vi "Enqueue Message.vi"(6 "Prioritary message":bool, 7 "QueueName":string, 8 "error in":errorcluster, 9 "Data":variant, 10 "Message":string, 11 "Queue":refnum<queue>) -> (0 "error out":errorcluster, 3 "Queue dup.":refnum<queue>)   [LabVIEW 2016, in "Message Queue.lvlib"]
doc: "Pour un message normal, placer le message à la fin de la file d'attente. Pour un message prioritaire, l'ajouter au début de la file."
uses:
  Message Queue.lvlib
  Message Cluster.ctl
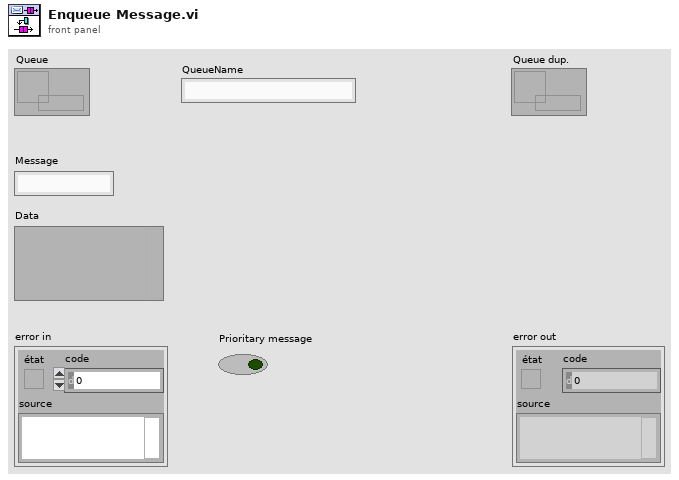
[diagram p1: front panel]
types:
  T1 = typedef "Message Queue.lvlib/Message Cluster.ctl" = cluster{"Message":string, "Données de message":variant}
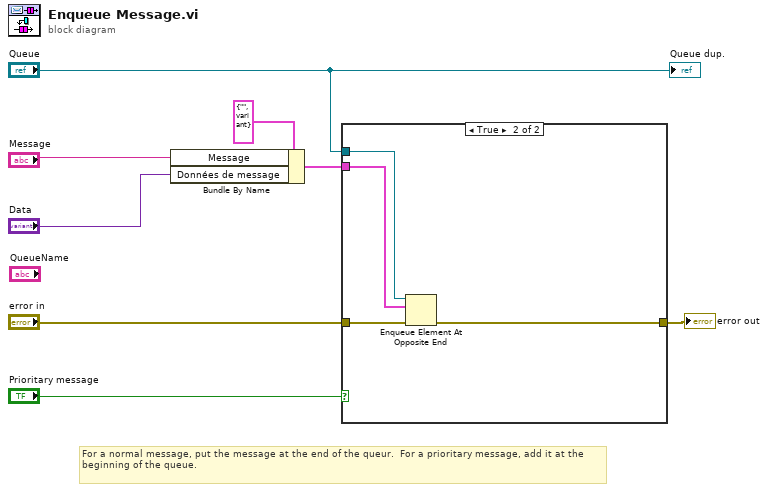
[diagram p0: block diagram]
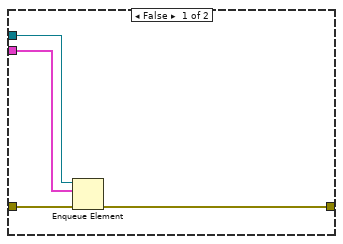
[diagram p2: hidden frame]
diagram:
  # "For a normal message, put the message at the end of the queur.  For a prioritary message, add it at the beginning of the queue."
  n1 = Bundle By Name(cluster=T1 {"Message"="", "Données de message"=variant} ("Cluster Message"), "Message"="Message", "Données de message"="Data") -> (w1:T1)
  n2 = case shown="True" "Prioritary message" {
    tunnel: "error in" -> [w12 w16]
    tunnel: [w11 w15] -> w3
    tunnel: "Queue" -> [w10 w14]
    tunnel: w1 -> [w9 w13]
    frame False {
      n3 = Enqueue Element(queue=w10, element=w9, error in (no error)=w12) -> (error out=w11:errorcluster)  [unwired: 1 in, 2 out]
    }
    frame True {
      n4 = Enqueue Element At Opposite End(queue=w14, element=w13, error in (no error)=w16) -> (error out=w15:errorcluster)  [unwired: 1 in, 2 out]
    }
  }
  "error out" <- w3
  "Queue dup." <- "Queue"
